vi "Save Submission.vi"(7 "Processing in":refnum<class "Processing.lvclass">, 8 "Challenge":refnum<class "Challenge.lvclass">, 9 "User":refnum<class "SOL User.lvclass">, 10 "File Path":path, 11 "Submit":refnum<class "Submit.lvclass">) -> (0 "error out":errorcluster, 5 "Processing out":refnum<class "Processing.lvclass">)   [LabVIEW 2020, in "Summer of LabVIEW.lvlib" / "Submit.lvclass"]
uses:
  Submit.lvclass
  <vilib>/IlluminatedG/IG HTTP Server/HTTP Server/Processing/Processing.lvclass
  Challenge/Challenge.lvclass
  SOL User/SOL User.lvclass
  Submission DB/Submission DB.lvclass
  <vilib>/IlluminatedG/IG HTTP Server/HTTP Server/Processing/Processing.lvclass/Processing.ctl
  Submit.lvclass/Submit.ctl
  fb2f95b6-9919-4798-a420-4d44da99c8cb.vi
  fb2f95b6-9919-4798-a420-4d44da99c8cb.vi/9528e9df-aefc-4ce0-9221-106a337fd3b6.vi
  <vilib>/IlluminatedG/IG HTTP Server/HTTP Server/Values/Get Arg Map.vi
  <vilib>/Utility/error.llb/Error Cluster From Error Code.vi
  Submission/Submission.lvclass
  <vilib>/IlluminatedG/IG HTTP Utils/HTTP Utils/Response/Response.lvclass
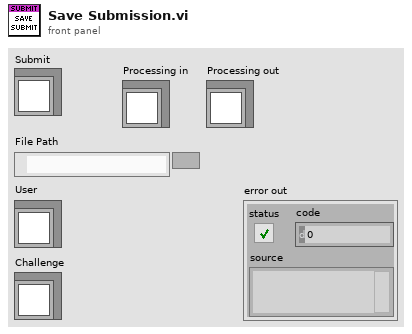
[diagram p1: front panel]
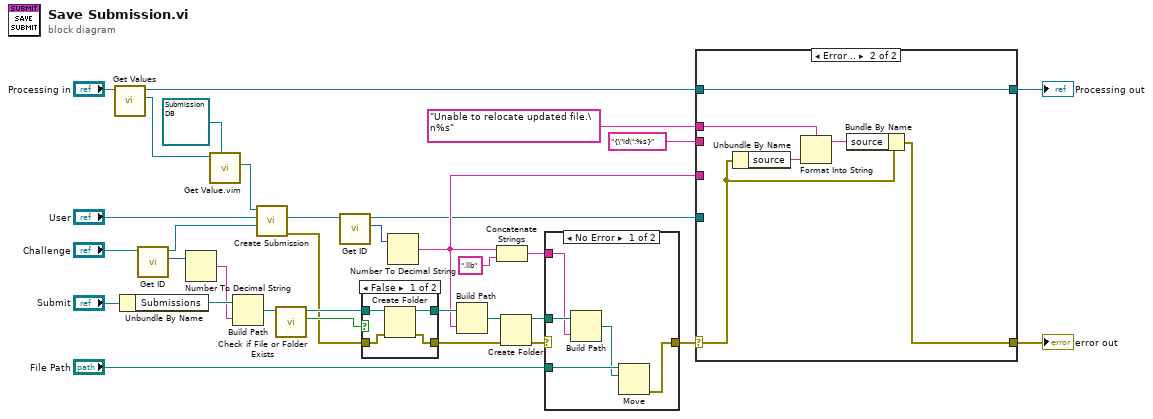
[diagram p0: block diagram]
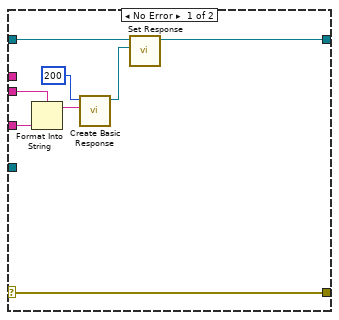
[diagram p2: hidden frame]
diagram:
  n1 = call <vilib>:"Get Values.vi"("Processing in"="Processing in") -> ("Values"=w32:refnum<class "Values.lvclass">, "Processing out"=w9:refnum<class "Processing.lvclass">)  [unwired: 9 in]
  n2 = Unbundle By Name("Submit") -> ("Submissions"=w23:path)
  n3 = call "Get ID.vi"("Challenge in"="Challenge") -> ("ID"=w24:i64, "Challenge out"=w25:refnum<class "Challenge.lvclass">)  [unwired: 9 in]
  n4 = Number To Decimal String(number=w24) -> (decimal integer string=w22:string)  [unwired: 1 in]
  n5 = call "Get Value.vim"("Type / Server / Service (String)"=refnum<class "Submission DB.lvclass"> refnum ("SOL:Submission DB.lvclass"), "Arguments in"=w32) -> ("Value"=w30:refnum<class "Submission DB.lvclass">)  [unwired: 7 in, 2 out]
  n6 = Build Path(base path=w23, name or relative path=w22) -> (appended path=w21:path)
  n7 = call "Create Submission.vi"("Challenge"=w25, "User"="User", "Submission DB in"=w30) -> ("error out"=w2:errorcluster, "Submission"=w28:refnum<class "Submission.lvclass">)  [unwired: 6 in, 1 out]
  n8 = call <vilib>:"Check if File or Folder Exists.vi"("path"=w21) -> ("file or folder exists?"=w20:bool, "dup path"=w19:path)  [unwired: 8 in, 1 out]
  n9 = call "Get ID.vi"("Submission in"=w28) -> ("ID"=w17:i64, "Submission out"=w3:refnum<class "Submission.lvclass">)  [unwired: 9 in]
  n10 = case shown="False" w20 {
    tunnel: w19 -> [w37 w39]
    tunnel: [w36 w39] -> w18
    tunnel: [w35 w38] -> w15
    tunnel: w2 -> [w34 w38]
    frame False {
      n11 = Create Folder(path (use dialog)=w37, error in=w34) -> (created path=w36:path, error out=w35:errorcluster)  [unwired: 1 in, 1 out]
    }
    frame True {
    }
  }
  n12 = Number To Decimal String(number=w17) -> (decimal integer string=w7:string)  [unwired: 1 in]
  n13 = Build Path(base path=w18, name or relative path=w7) -> (appended path=w16:path)
  n14 = Concatenate Strings(w7, ".llb" ("string")) -> (w11:string)
  n15 = Create Folder(path (use dialog)=w16, error in=w15) -> (created path=w12:path, error out=w10:errorcluster)  [unwired: 1 in, 1 out]
  n16 = case shown="No Error" w10 {
    selector: w10 -> [_ w45]
    tunnel: "File Path" -> [w44 _]
    tunnel: w12 -> [w43 _]
    tunnel: w11 -> [w42 _]
    tunnel: [w40 w45] -> w8
    frame No Error {
      n17 = Build Path(base path=w43, name or relative path=w42) -> (appended path=w41:path)
      n18 = Move(source path=w44, 10:w41) -> (error out=w40:errorcluster)  [unwired: 3 in, 2 out]
    }
    frame Error {
    }
  }
  n19 = case shown="Error .." w8 {
    selector: w8 -> [w46 w57]
    tunnel: w9 -> [w49 w55]
    tunnel: w7 -> [w52 _]
    tunnel: "{\"id\":%s}" -> [w51 _]
    tunnel: [w47 w55] -> w5
    tunnel: "Unable to relocate updated file.\n%s" ("Payload") -> [_ w59]
    tunnel: w3 -> [_ _]
    tunnel: [w46 w54] -> w1
    frame No Error {
      n20 = Format Into String(format string=w51, w52) -> (resulting string=w50:string)  [unwired: 2 in, 1 out]
      n21 = call <vilib>:"Create Basic Response.vi"("Payload"=w50, "Status Code"=u16 200) -> ("Response out"=w48:refnum<class "Response.lvclass">)  [unwired: 8 in, 1 out]
      n22 = call <vilib>:"Set Response.vi"("Response"=w48, "Processing in"=w49) -> ("Processing out"=w47:refnum<class "Processing.lvclass">)  [unwired: 9 in]
    }
    frame Error {
      n23 = Unbundle By Name(w57) -> ("source"=w58:string)
      n24 = Format Into String(format string=w59, w58) -> (resulting string=w56:string)  [unwired: 2 in, 1 out]
      n25 = Bundle By Name(cluster=w57, "source"=w56) -> (w54:errorcluster)
    }
  }
  "Processing out" <- w5
  "error out" <- w1
